vi "Translate_PolarVector.vi"(7 "Translation Type":T1, 8 "error in (no error)":errorcluster, 11 "CartesianVector in":refnum<class "CartesianVector.lvclass">) -> (0 "error out":errorcluster, 3 "CartesianVector out":refnum<class "CartesianVector.lvclass">)   [LabVIEW 2011, in "CartesianVector.lvclass"]
uses:
  CartesianVector.lvclass
  TypeDefs/TranslationType.ctl
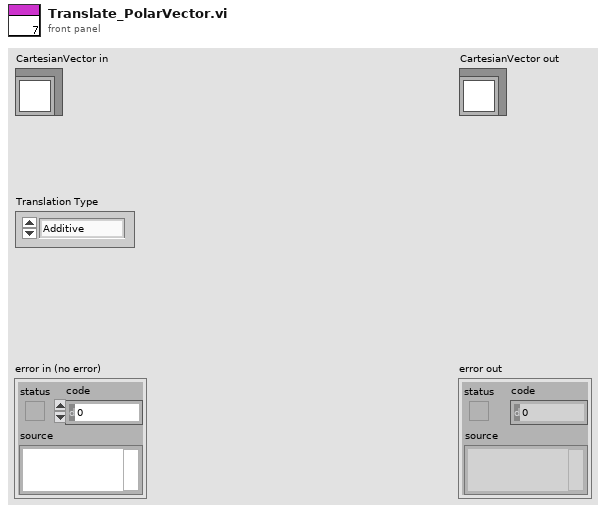
[diagram p1: front panel]
types:
  T1 = typedef "TranslationType.ctl" = enum16{"Additive", "Subtractive"}
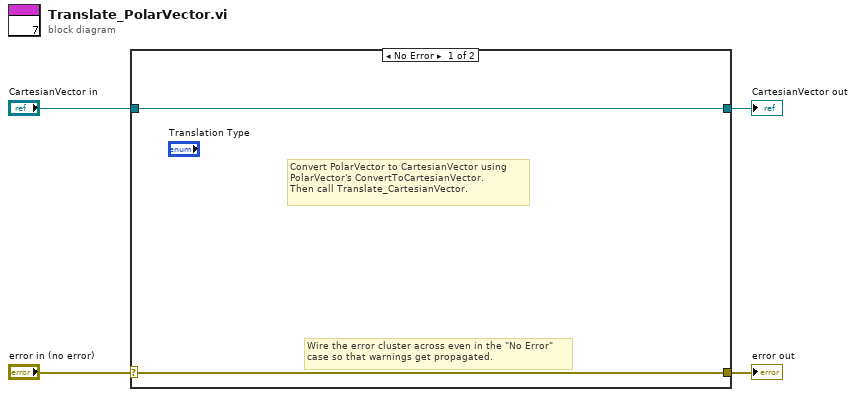
[diagram p0: block diagram]
diagram:
  n1 = case shown="No Error" "error in (no error)" {
    selector: "error in (no error)" -> [w5 w8]
    tunnel: [w5 w8] -> w3
    tunnel: [w6 w7] -> w1
    tunnel: "CartesianVector in" -> [w6 w7]
    frame No Error {
      # "Convert PolarVector to CartesianVector using\nPolarVector's ConvertToCartesianVector.\nThen call Translate_CartesianVector."
      # "Wire the error cluster across even in the \"No Error\"\ncase so that warnings get propagated."
    }
    frame Error {
    }
  }
  "error out" <- w3
  "CartesianVector out" <- w1
